vi "PH_DataViewer.set Current Meas GUI Elements.vi"(2 "Current Meas'":T1[](array[typedef]), 5 "Version":u8) -> (10 "Snapshot: Date":string, 11 "Data":waveform(dbl)[][](array[waveform]), 12 "Snapshot: Time":string, 13 "Ignore Timestamp":bool, 14 "Power Unit List":string[](array[string]), 15 "index":i32, 16 "PU Name":string, 17 "Graph Data":waveform(dbl)[](array[waveform]), 18 "X Scale.Format & Precision:Precision":u8, 19 "index of element":i32)   [LabVIEW 2014, in "PH_DataViewer.lvlib"]
doc: "This VI prepares the information to be indicated."
uses:
  PH_DataViewer.lvlib
  PH_CurrentMeas.Data.ctl
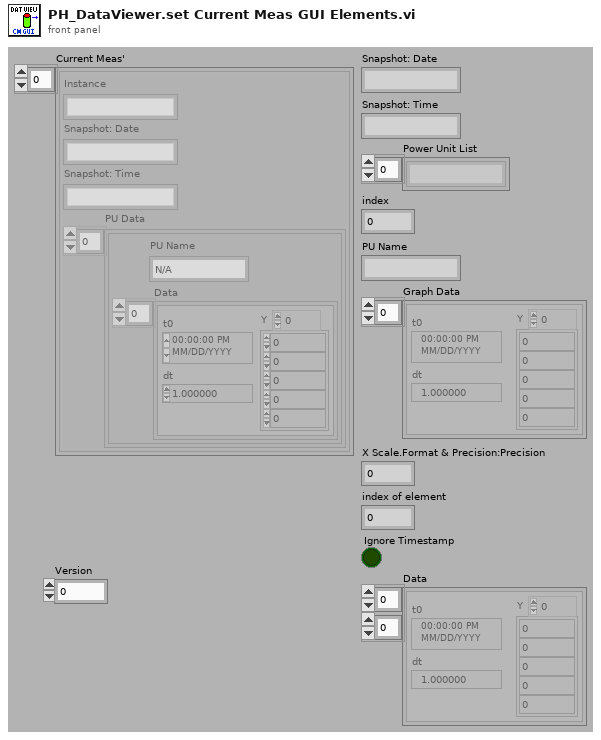
[diagram p1: front panel]
types:
  T1 = typedef "PH_DataViewer.lvlib/PH_CurrentMeas.Data.ctl" = cluster{"Instance":string, "Snapshot: Date":string, "Snapshot: Time":string, "PU Data":cluster{"Data":waveform(dbl)[], "PU Name":string}[]}
  T2 = cluster{"Data":waveform(dbl)[], "PU Name":string}[]
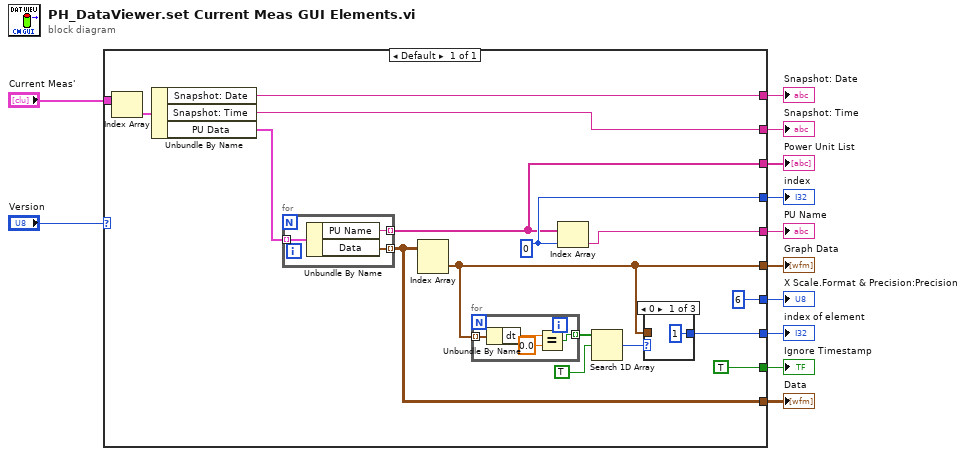
[diagram p0: block diagram]
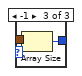
[diagram p3: hidden frame]
diagram:
  n1 = case shown="Default" "Version" {
    tunnel: [w28] -> w12
    tunnel: [TRUE ("Ignore Timestamp")] -> w11
    tunnel: [w26] -> w10
    tunnel: [w25] -> w9
    tunnel: [w23] -> w8
    tunnel: [w22] -> w7
    tunnel: [u8 6 ("X Scale.Format & Precision:Precision")] -> w6
    tunnel: [w18] -> w5
    tunnel: [w16] -> w4
    tunnel: [w15] -> w3
    tunnel: "Current Meas'" -> [w13]
    frame Default {
      w28 = 0 ("index")
      n2 = Index Array(array=w13) -> (element=w14:T1)  [unwired: 1 in]
      n3 = Unbundle By Name(w14) -> ("Snapshot: Date"=w15:string, "Snapshot: Time"=w16:string, "PU Data"=w17:T2)
      n4 = for {
        tunnel: w17 -> [w39] mode=indexing
        tunnel: [w38] -> w22 mode=indexing
        tunnel: [w37] -> w18 mode=indexing
        n5 = Unbundle By Name(w39) -> ("PU Name"=w38:string, "Data"=w37:waveform(dbl)[])
      }
      n6 = Index Array(array=w18) -> (element=w26:waveform(dbl)[])  [unwired: 2 in]
      n7 = for {
        tunnel: w26 -> [w36] mode=indexing
        tunnel: [w33] -> w20 mode=indexing
        n8 = Unbundle By Name(w36) -> ("dt"=w35:dbl)
        n9 = Equal?(x=w35, y=0.0) -> (x = y?=w33:bool)
      }
      n10 = Index Array(array=w22, index=w28) -> (element=w23:string)
      n11 = Search 1D Array(1D array=w20, element=TRUE) -> (index of element=w24:i32)  [unwired: 1 in]
      n12 = case shown="0" w24 {
        selector: w24 -> [_ w30 _]
        tunnel: w26 -> [_ _ w32]
        tunnel: [1 ("index of element") w30 w31] -> w25
        frame 0 {
        }
        frame Default {
        }
        frame -1 {
          n13 = Array Size(array=w32) -> (size(s)=w31:i32)
        }
      }
    }
  }
  "index" <- w12
  "Ignore Timestamp" <- w11
  "Graph Data" <- w10
  "index of element" <- w9
  "PU Name" <- w8
  "Power Unit List" <- w7
  "X Scale.Format & Precision:Precision" <- w6
  "Data" <- w5
  "Snapshot: Time" <- w4
  "Snapshot: Date" <- w3
